vi "Write Execute_.vi"(8 "error in (no error)":errorcluster, 10 "Execute?":bool=TRUE, 11 "Beep Msg in":refnum<class "Beep Msg.lvclass">) -> (0 "error out":errorcluster, 3 "Beep Msg out":refnum<class "Beep Msg.lvclass">)   [LabVIEW 2016, in "CS++BeepActor.lvlib" / "Beep Msg.lvclass"]
uses:
  Beep Msg.lvclass
  Beep Msg.lvclass/Beep Msg.ctl
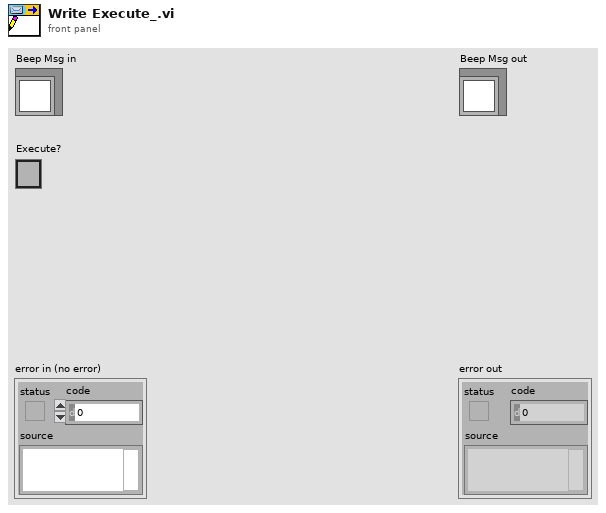
[diagram p1: front panel]
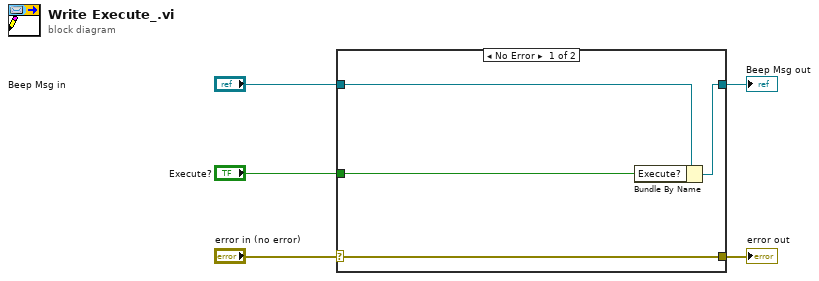
[diagram p0: block diagram]
diagram:
  n1 = case shown="No Error" "error in (no error)" {
    selector: "error in (no error)" -> [w9 w10]
    tunnel: [w9 w10] -> w4
    tunnel: [w7 w11] -> w2
    tunnel: "Beep Msg in" -> [w8 w11]
    tunnel: "Execute?" -> [w6 _]
    frame No Error {
      n2 = Bundle By Name(cluster=w8, "Execute?"=w6) -> (w7:refnum<class "Beep Msg.lvclass">)
    }
    frame Error {
    }
  }
  "error out" <- w4
  "Beep Msg out" <- w2
